vi "Remove Process from App.vi"(8 "error in (no error)":errorcluster, 10 "String":string, 11 "Application in":refnum<class "Application.lvclass">) -> (0 "error out":errorcluster, 2 "Process":refnum<class "Process.lvclass">, 3 "Application out":refnum<class "Application.lvclass">)   [LabVIEW 2020, in "Application.lvclass"]
uses:
  Application.lvclass
  C:/Users/anton/Documents/GitHub/Triarc-Framework/source/Framework/Process/Process.lvclass
  Process/Process.lvclass
  Process/Process.lvclass/Process.ctl
  Process/Public/Lifecycle/Get Lifecycle State.vi
  Process/Private/SubVIs/Enqueue Request Message.vi
  <vilib>/Utility/error.llb/Clear Errors.vi
  <vilib>/Utility/error.llb/Error Cluster From Error Code.vi
  Process/Private/SubVIs/Wait for Response Message.vi
  C:/Users/anton/Documents/GitHub/Triarc-Framework/source/Framework/Base/Base.lvclass
  C:/Users/anton/Documents/GitHub/Triarc-Framework/source/Framework/Error Handler Interface/Error Handler Interface.lvclass
  C:/Users/anton/Documents/GitHub/Triarc-Framework/source/Framework/Logging/Logging.lvclass
  C:/Users/anton/Documents/GitHub/Triarc-Framework/source/Framework/Application/Application.lvclass
  C:/Users/anton/Documents/GitHub/Triarc-Framework/source/Framework/Async Handler/Async Handler.lvclass
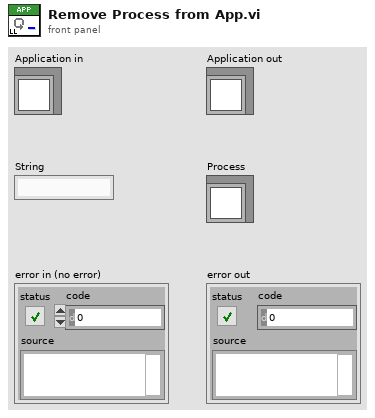
[diagram p1: front panel]
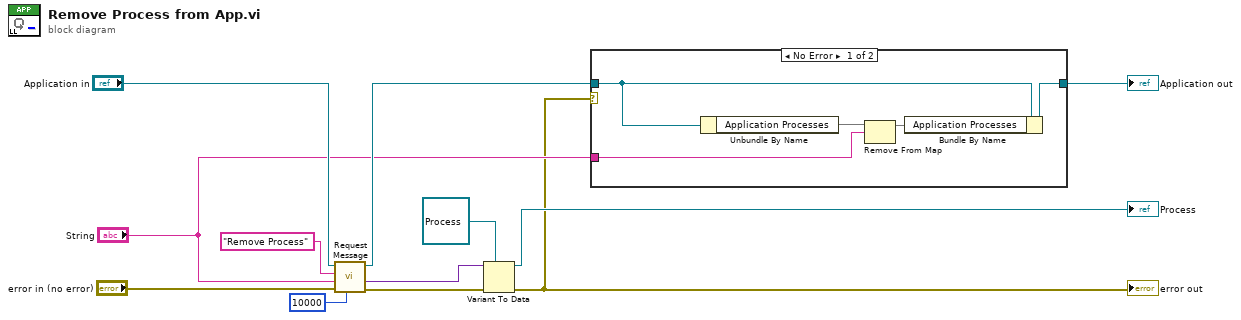
[diagram p0: block diagram]
diagram:
  n1 = call "Request Message.vi"("timeout in ms (-1)"=10000, "error in (no error)"="error in (no error)", "Request Message Data"="String", "Request Message"="Remove Process", "Process In"="Application in") -> ("error out"=w9:errorcluster, "Response Message Data"=w7:variant, "Process Out"=w4:refnum<class "Application.lvclass">)  [unwired: 2 in, 2 out]
  n2 = Variant To Data(error in=w9, type=refnum<class "Process.lvclass"> refnum ("Rig Process"), Variant=w7) -> (data=→"Process":refnum<class "Process.lvclass">, error out=w1:errorcluster)
  "error out" <- w1
  n3 = case shown="No Error" w1 {
    tunnel: w4 -> [w17 w18]
    tunnel: "String" -> [w15 _]
    tunnel: [w14 w18] -> w2
    frame No Error {
      n4 = Unbundle By Name(w17) -> ("Application Processes"=w16:map{string, refnum<class "Process.lvclass">})
      n5 = Remove From Map(10:w15, 11:w16) -> (3:w13:map{string, refnum<class "Process.lvclass">})  [unwired: 2 out]
      n6 = Bundle By Name(cluster=w17, "Application Processes"=w13) -> (w14:refnum<class "Application.lvclass">)
    }
    frame Error {
    }
  }
  "Application out" <- w2
